vi "Siglent SDG X Series Standard Waveform-APP.vi"() -> ()   [LabVIEW 2020]
doc: "This example shows how to generate a standard waveform."
uses:
  <instrlib>/Siglent SDG X Series/Siglent SDG X Series.lvlib
panel:
  in  "Low Volts":dbl
  in  "High Volts":dbl=5.0
  in  "OK":bool
  in  "Duty Cycle (50.0%)":dbl=98.0 min=20.0 max=99.0 format="%.1g"
  out "Amplitude (1.0 Vpp)":dbl=5.0 format="%#.3f"
  in  "VISA resource name":refnum<visa-resource-name>
  out "DC Offset (0.00 V)":dbl=-2.5
  in  "Frequency (1000 Hz)":dbl=1.0 format="%#.6g"
  in  "Channel (1:Channel 1)":i32(ring)=1 items=["Channel 1"=1, "Channel 2"=2]
  in  "Waveform Function (0: Sine)":u16(ring)=1 items=["Sine", "Square", "Triangle", "DC", "Pulse", "Arb"]
  # "WARNING. RUN ONLY WHEN LASER IS SHUTTERED"
  # "(c) 2017 SIGLENT TECHNOLOGIES CO.,LTD. ALL RIGHTS RESERVED."
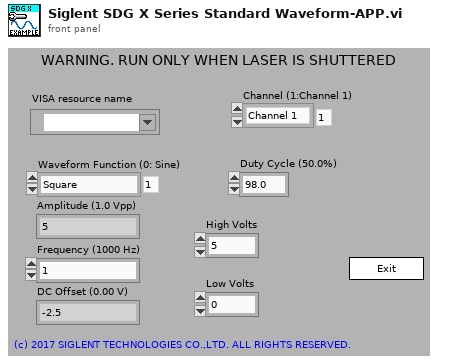
[diagram p1: front panel]
types:
  T1 = enum32{"Invalid", "Standard", "Closed", "Hidden", "Minimized", "Maximized"}
  T2 = enum32{"invalid app kind", "Development System", "Run Time System", "Student Edition", "Embedded LabVIEW", "Evaluation", "Custom"}
  T3 = cluster{"Core":cluster{"Current VI Reference":refnum<vi>, "Close Panel on Exit?":bool}, "VISA resource name":refnum<visa-resource-name>, "Channel (1:Channel 1)":i32}
  T4 = cluster{"Current VI Reference":refnum<vi>, "Close Panel on Exit?":bool}
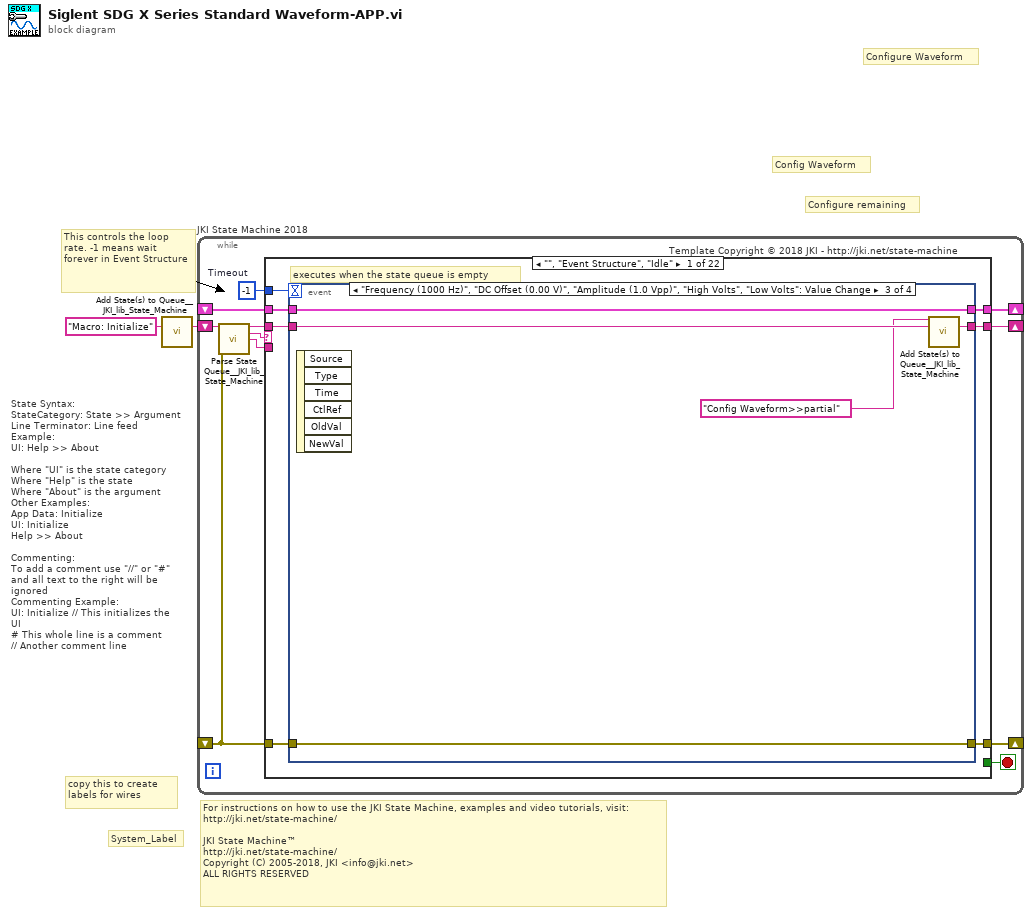
[diagram p0: block diagram]
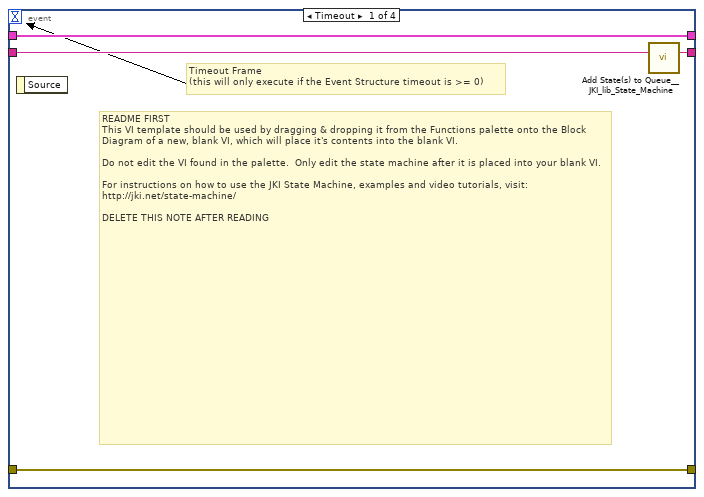
[diagram p2: hidden frame]
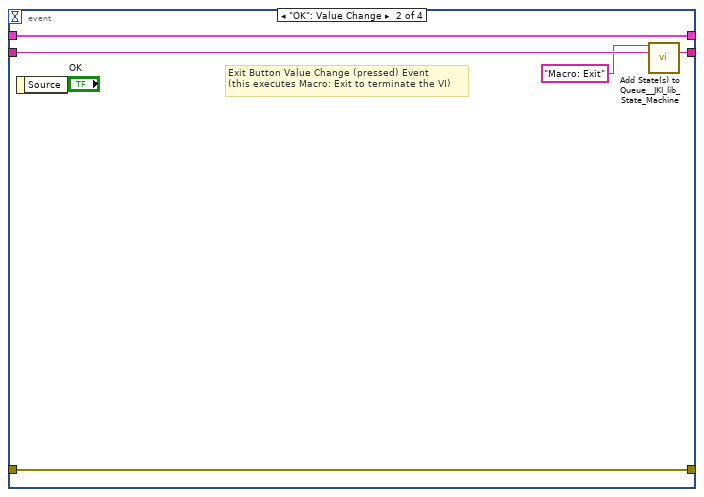
[diagram p3: hidden frame]
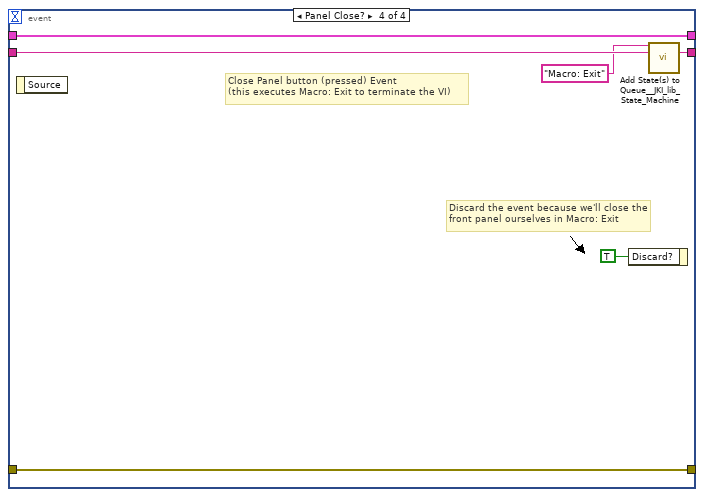
[diagram p4: hidden frame]
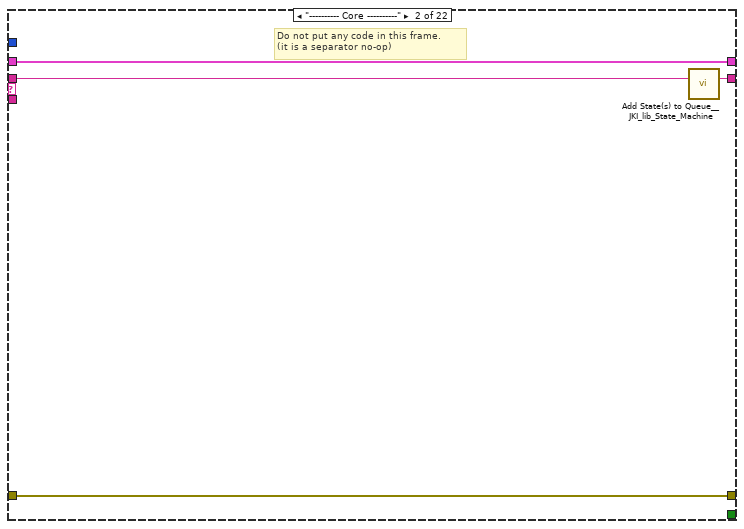
[diagram p5: hidden frame]
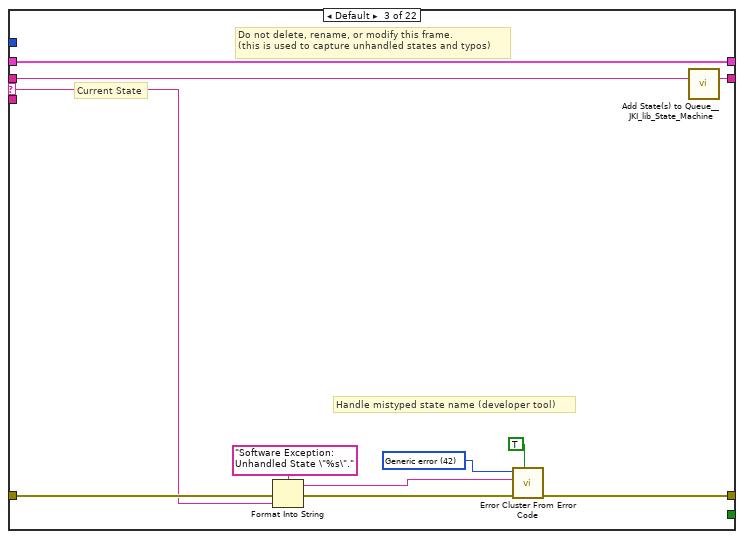
[diagram p6: hidden frame]
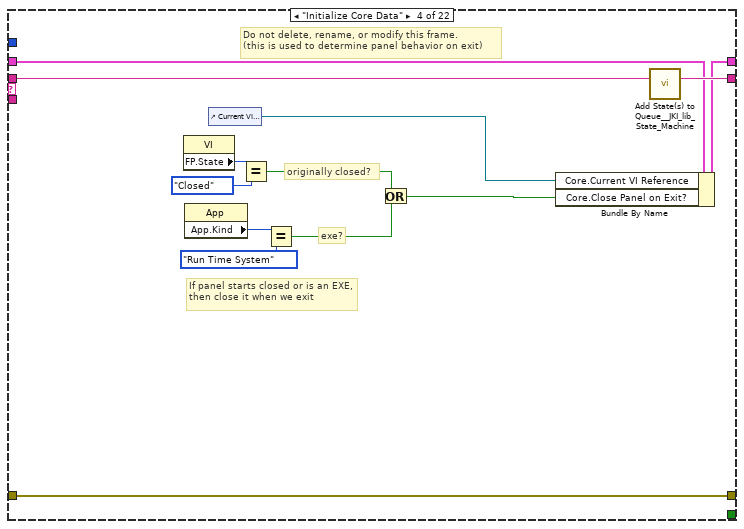
[diagram p7: hidden frame]
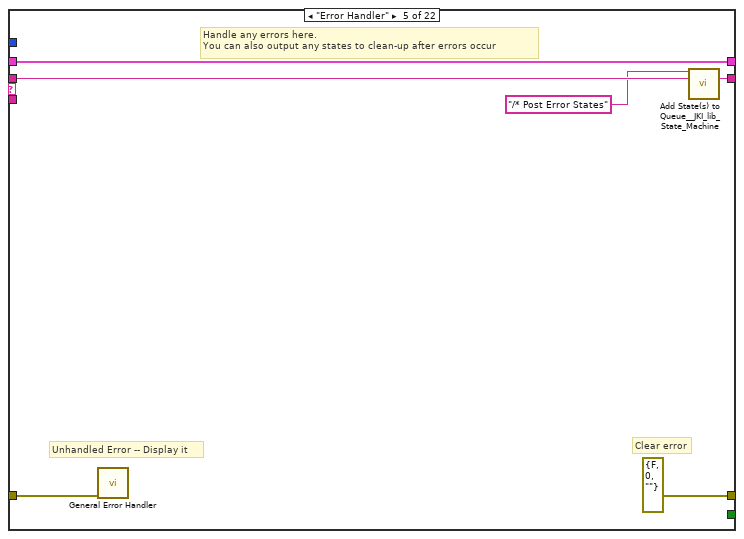
[diagram p8: hidden frame]
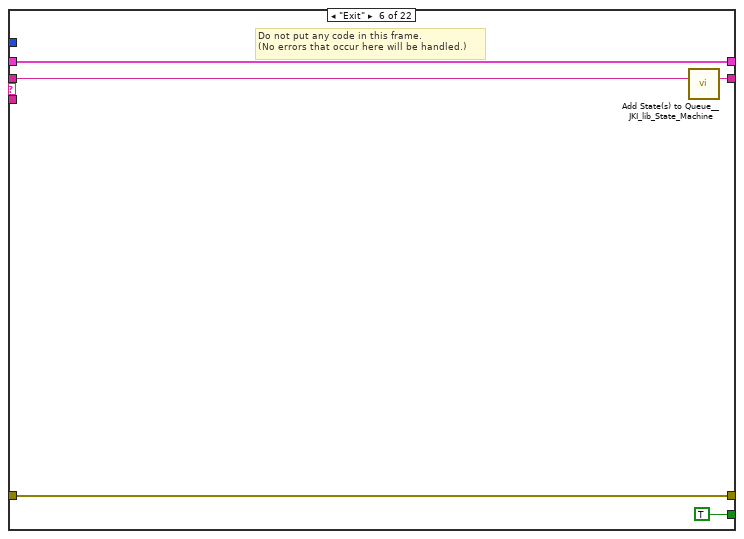
[diagram p9: hidden frame]
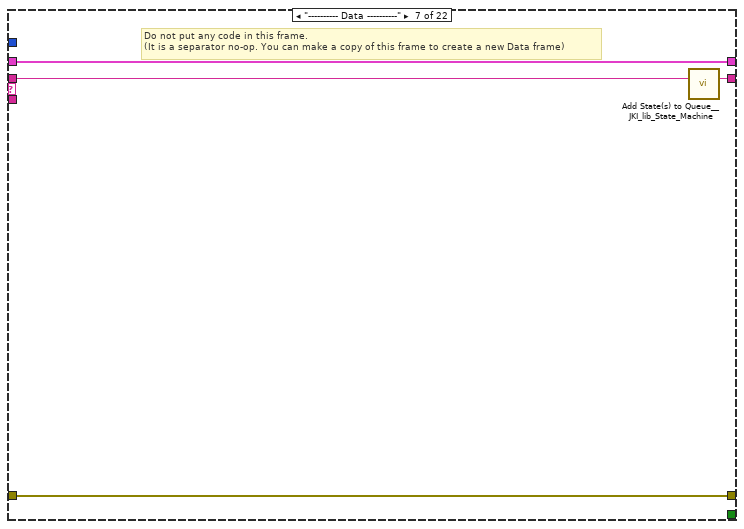
[diagram p10: hidden frame]
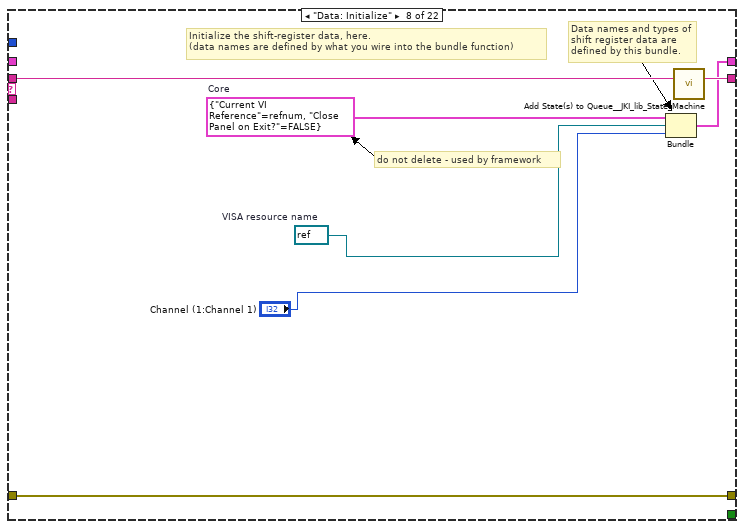
[diagram p11: hidden frame]
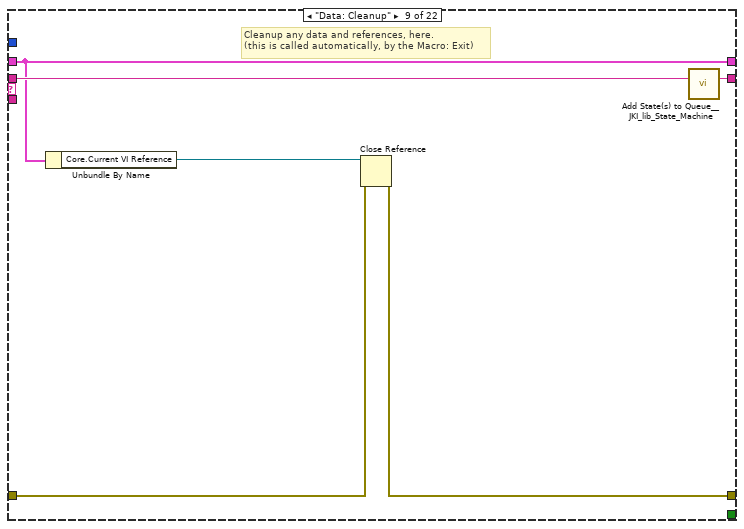
[diagram p12: hidden frame]
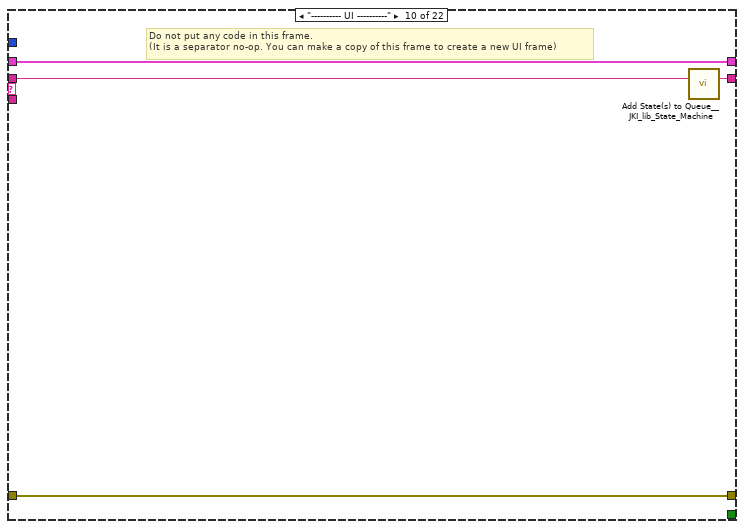
[diagram p13: hidden frame]
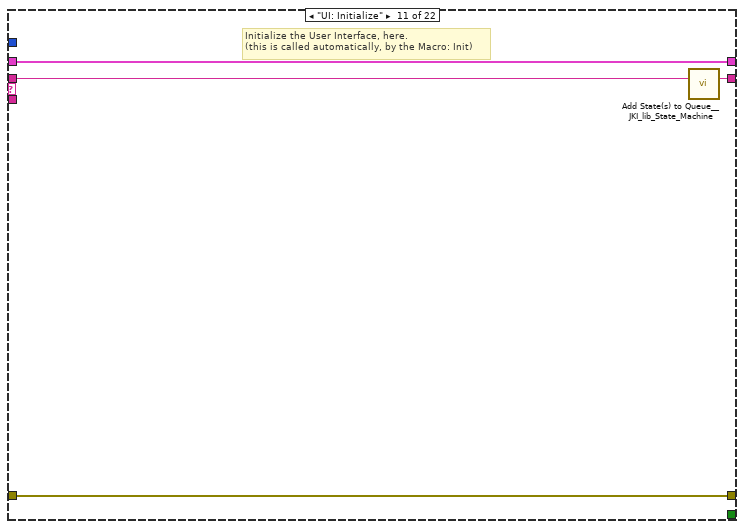
[diagram p14: hidden frame]
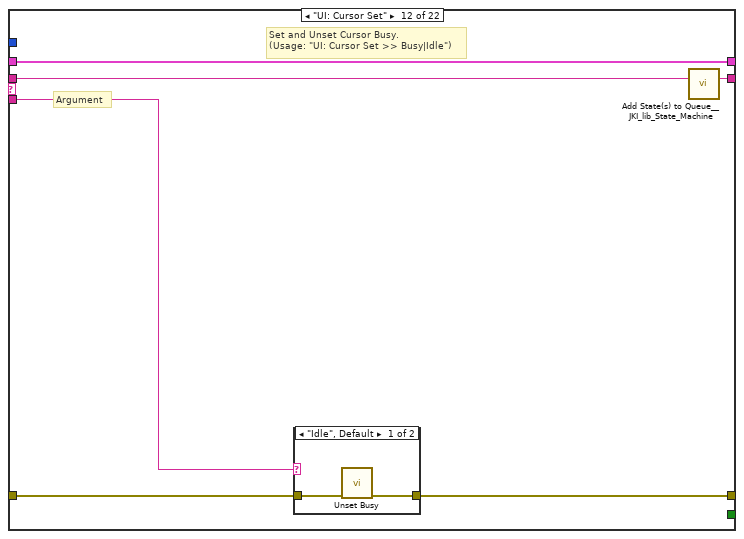
[diagram p15: hidden frame]
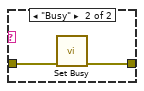
[diagram p16: hidden frame]
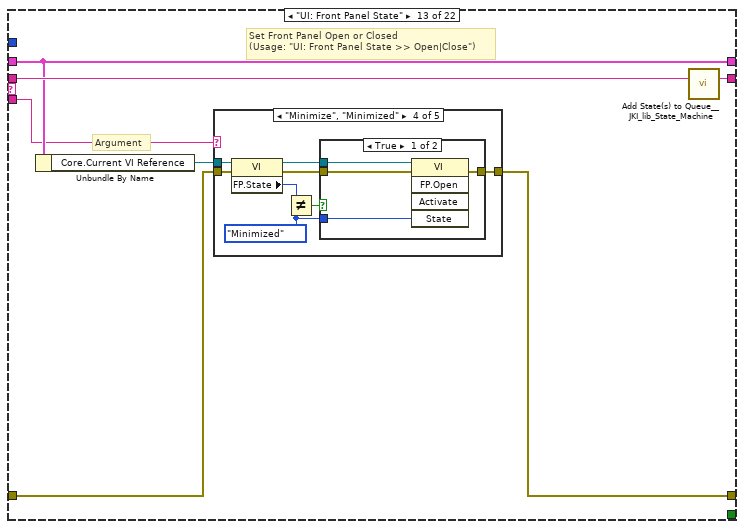
[diagram p17: hidden frame]
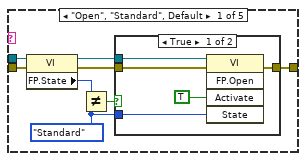
[diagram p18: hidden frame]
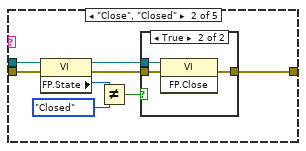
[diagram p20: hidden frame]
diagram:
  # "Configure remaining"
  # "Config Waveform"
  # "For instructions on how to use the JKI State Machine, examples and video tutorials, visit:\nhttp://jki.net/state-machine/\n\nJKI State Machine™\nhttp://jki.net/state-machine/\nCopyright (C) 2005-2018, JKI <info@jki.net>\nALL RIGHTS RESERVED"
  # "State Syntax:\nStateCategory: State >> Argument\nLine Terminator: Line feed\nExample:\nUI: Help >> About\n\nWhere \"UI\" is the state category\nWhere \"Help\" is the state\nWhere \"About\" is the argument\nOther Examples:\nApp Data: Initialize\nUI: Initialize\nHelp >> About\n\nCommenting:\nTo add a comment use \"//\" or \"#\" and all text to the right will be ignored\nCommenting Example:\nUI: Initialize // This initializes the UI\n# This whole line is a comment\n// Another comment line"
  # "copy this to create labels for wires"
  # "This controls the loop rate. -1 means wait forever in Event Structure"
  # "System_Label"
  # "Configure Waveform"
  n1 = call <vilib>:"Add State(s) to Queue__JKI_lib_State_Machine.vi"("State(s) in (\"\")"="Macro: Initialize") -> ("States Out"=w2:string)  [unwired: 14 in]
  n2 = while "JKI State Machine 2018" {
    shift-right: [w6] -> _
    shift-left: _ -> [w5]
    shift-right: [w9] -> _
    shift-left: _ -> [w3]
    shift-right: [w8] -> _
    shift-left: w2 -> [w10]
    stop <- w7 stop-if-true
    w4 = -1  # Timeout
    # "Template Copyright © 2018 JKI - http://jki.net/state-machine"
    n3 = call <vilib>:"Parse State Queue__JKI_lib_State_Machine.vi"("State Queue"=w10, "Error In (no error)"=w3) -> ("Remaining States"=w12:string, "Current State"=w13:string, "Arguments"=w11:string)  [unwired: 11 in]
    n4 = case shown="\"\", \"Event Structure\", \"Idle\"" w13 {
      selector: w13 -> [_ _ w45 _ _ _ _ _ _ _ _ _ _ _ _ _ _ _ _ _ _ _]
      tunnel: w12 -> [w20 w44 w49 w68 w74 w79 w83 w90 w96 w100 w104 w110 w121 w190 w195 w205 w209 w223 w243 w249 w269 w277]
      tunnel: w11 -> [_ _ _ _ _ _ _ _ _ _ _ w105 w115 _ _ _ _ w214 _ _ _ _]
      tunnel: w5 -> [w18 w41 w47 w61 w71 w77 w80 _ w91 w97 w102 w108 w117 w187 w192 w202 w206 w217 w240 w247 w267 w272]
      tunnel: [w17 w42 w51 w65 errorcluster {"status"=FALSE, "code"=0, "source"=""} ("error out") w76 w81 w87 w92 w98 w101 w106 w118 w188 w193 w203 w207 w218 w241 w244 w252 w275] -> w9
      tunnel: w3 -> [w16 w42 w50 w65 w70 w76 w81 w87 w93 w98 w101 w107 w119 w188 w193 w203 w207 w219 w241 w245 w253 w275]
      tunnel: [w19 w43 w48 w67 w73 w78 w82 w89 w95 w99 w103 w109 w120 w189 w194 w204 w208 w222 w242 w248 w268 w276] -> w8
      tunnel: [_ _ _ _ _ TRUE _ _ _ _ _ _ _ _ _ _ _ _ _ _ _ _] -> w7
      tunnel: [w15 w41 w47 w66 w71 w77 w80 w88 w91 w97 w102 w108 w117 w187 w192 w202 w206 w217 w240 w247 w267 w270] -> w6
      tunnel: w4 -> [w14 _ _ _ _ _ _ _ _ _ _ _ _ _ _ _ _ _ _ _ _ _]
      frame "", "Event Structure", "Idle" {
        # "executes when the state queue is empty"
        n5 = event shown="[2] \"Frequency (1000 Hz)\", \"DC Offset (0.00 V)\", \"Amplitude (1.0 Vpp)\", \"High Volts\", \"Low Volts\": Value Change" {
          selector: _ -> [_ _ _ _]
          dyn-events: _ -> [_ _ _ _]
          timeout: w14 -> [_ _ _ _]
          tunnel: w20 -> [w24 w29 w34 w40]
          tunnel: [w23 w28 w33 w39] -> w19
          tunnel: w18 -> [w21 w26 w31 w37]
          tunnel: [w22 w27 w32 w38] -> w17
          tunnel: w16 -> [w22 w27 w32 w38]
          tunnel: [w21 w26 w31 w37] -> w15
          event Timeout {
            # "README FIRST\nThis VI template should be used by dragging & dropping it from the Functions palette onto the Block Diagram of a new, blank VI, which will place it's contents into the blank VI.\n\nDo not edit the VI found in the palette.  Only edit the state machine after it is placed into your blank VI.\n\nFor instructions on how to use the JKI State Machine, examples and video tutorials, visit:\nhttp://jki.net/state-machine/\n\nDELETE THIS NOTE AFTER READING"
            # "Timeout Frame\n(this will only execute if the Event Structure timeout is >= 0)"
            n6 = event-data() -> ()  [unwired: 1 in, 1 out]
            n7 = call <vilib>:"Add State(s) to Queue__JKI_lib_State_Machine.vi"("State(s) in (\"\")"=w24) -> ("States Out"=w23:string)  [unwired: 14 in]
          }
          event "OK": Value Change {
            # "Exit Button Value Change (pressed) Event\n(this executes Macro: Exit to terminate the VI)"
            n8 = event-data() -> ()  [unwired: 1 in, 1 out]
            n9 = call <vilib>:"Add State(s) to Queue__JKI_lib_State_Machine.vi"("State(s) in Front (\"\")"="Macro: Exit", "State(s) in (\"\")"=w29) -> ("States Out"=w28:string)  [unwired: 13 in]
          }
          event "Frequency (1000 Hz)", "DC Offset (0.00 V)", "Amplitude (1.0 Vpp)", "High Volts", "Low Volts": Value Change {
            n10 = event-data() -> ()  [unwired: 1 in, 6 out]
            n11 = call <vilib>:"Add State(s) to Queue__JKI_lib_State_Machine.vi"("State(s) in Front (\"\")"="Config Waveform>>partial", "State(s) in (\"\")"=w34) -> ("States Out"=w33:string)  [unwired: 13 in]
          }
          event Panel Close? {
            # "Discard the event because we'll close the front panel ourselves in Macro: Exit"
            # "Close Panel button (pressed) Event\n(this executes Macro: Exit to terminate the VI)"
            n12 = event-data() -> ()  [unwired: 1 in, 1 out]
            n13 = event-data("Discard?"=TRUE) -> ()  [unwired: 1 in, 1 out]
            n14 = call <vilib>:"Add State(s) to Queue__JKI_lib_State_Machine.vi"("State(s) in Front (\"\")"="Macro: Exit", "State(s) in (\"\")"=w40) -> ("States Out"=w39:string)  [unwired: 13 in]
          }
        }
      }
      frame "---------- Core ----------" {
        # "Do not put any code in this frame.\n(it is a separator no-op)"
        n15 = call <vilib>:"Add State(s) to Queue__JKI_lib_State_Machine.vi"("State(s) in (\"\")"=w44) -> ("States Out"=w43:string)  [unwired: 14 in]
      }
      frame Default {
        w54 = 42 items=["No error", "Argument error", "Memory is full", "Out of zone", "End of file", "File already open", "Generic file I/O error", "File not found", "File permission error", "Disk is full", "Duplicate path", "Too many files open", "System feature not enabled", "Resource file not found", "Cannot add resource", "Resource not found", "Image not found", "Image memory error", "Pen does not exist", "Config type invalid", "Config token not found", "Config parse error", "Config memory error", "Bad external code format", "Bad external code offset", "External code not present", "Null window", "Destroy window error", "Null menu", "Print aborted", "Bad print record", "Print driver error", "Windows error during printing", "Memory error during printing", "Print dialog error", "Generic print error", "Invalid device refnum", "Device not found", "Device parameter error", "Device unit error", "Cannot open device", "Device call aborted", "Generic error", "Cancelled by user", "Object ID too low", "Object ID too high", "Object not in heap", "Unknown heap", "Unknown object (invalid DefProc)", "Unknown object (DefProc not in table)", "Message out of range", "Invalid (null) method", "Unknown message", "Manager call not supported", "Bad address", "Network operation in progress", "Network operation timed out", "Connection is busy", "Network attribute not supported", "Network error", "Address in use", "System out of memory", "Connection aborted", "Connection refused", "Not connected", "Already connected", "Connection closed", "Initialization error (interapplication manager)", "Bad occurrence", "Wait on unbound occurrence handler", "Occurrence queue overflow", "Datalog type conflict", "Unused", "Unrecognized type (interapplication manager)", "Memory corrupt", "Failed to make temporary DLL", "Old CIN version", "Drag socket not found", "Failed to load drop-object", "Failed to register OLE object", "Failed to release OLE object", "Format specifier type mismatch", "Unknown format specifier", "Too few format specifiers", "Too many format specifiers", "Scan failed", "Newer CIN version", "Error converting to variant", "Runtime menu error", "Password tampered", "Variant attribute not found", "Incompatible variant data type", "Event data is not available", "Event Store is not present", "Occurrence is not found", "Event Queue is not created", "Event info is not available", "Refnum passed is NULL", "Error retrieving Class GUID", "Error retrieving CoClass GUID", "Error retrieving TypeLib GUID.", "Bad built application magic bytes.", "Specific driver is different from the specific driver associated with the Logical Name.", "There is no session opened to the class driver.", "Max Error", "MAX - Error with config objects", "MAX - Error loading configuration", "MAX - Group not supported"]
        # "Current State"
        # "Do not delete, rename, or modify this frame.\n(this is used to capture unhandled states and typos)"
        # "Handle mistyped state name (developer tool)"
        n16 = Format Into String(format string="Software Exception: Unhandled State \"%s\"." ("message"), error in=w50, w45) -> (resulting string=w53:string, error out=w52:errorcluster)  [unwired: 1 in]
        n17 = call <vilib>:"Error Cluster From Error Code.vi"("show call chain? (False)"=TRUE, "error in (no error)"=w52, "error message (\"\")"=w53, "error code (0)"=w54) -> ("error out"=w51:errorcluster)  [unwired: 5 in]
        n18 = call <vilib>:"Add State(s) to Queue__JKI_lib_State_Machine.vi"("State(s) in (\"\")"=w49) -> ("States Out"=w48:string)  [unwired: 14 in]
      }
      frame "Initialize Core Data" {
        # "Do not delete, rename, or modify this frame.\n(this is used to determine panel behavior on exit)"
        # "originally closed?"
        # "exe?"
        # "If panel starts closed or is an EXE, then close it when we exit"
        n19 = property class="VI"() -> ("FP.State"=w58:T1)  [unwired: 2 in, 2 out]
        n20 = property class="App"() -> ("App.Kind"=w64:T2)  [unwired: 2 in, 2 out]
        n21 = control-ref of="Current VI Reference"() -> (w59:refnum<vi>)
        n22 = Equal?(x=w58, y=T1."Closed" ("Front Panel Window:State")) -> (x = y?=w56:bool)
        n23 = Equal?(x=w64, y=T2."Run Time System" ("Application:Kind")) -> (x = y?=w62:bool)
        n24 = Or(x=w56, y=w62) -> (x .or. y?=w60:bool)
        n25 = Bundle By Name(cluster=w61, "Core.Current VI Reference"=w59, "Core.Close Panel on Exit?"=w60) -> (w66:T3)
        n26 = call <vilib>:"Add State(s) to Queue__JKI_lib_State_Machine.vi"("State(s) in (\"\")"=w68) -> ("States Out"=w67:string)  [unwired: 14 in]
      }
      frame "Error Handler" {
        # "Unhandled Error -- Display it"
        # "Handle any errors here.\nYou can also output any states to clean-up after errors occur"
        # "Clear error"
        n27 = call <vilib>:"General Error Handler.vi"("error in (no error)"=w70) -> ()  [unwired: 10 in, 5 out]
        n28 = call <vilib>:"Add State(s) to Queue__JKI_lib_State_Machine.vi"("State(s) in Front (\"\")"="/* Post Error States", "State(s) in (\"\")"=w74) -> ("States Out"=w73:string)  [unwired: 13 in]
      }
      frame "Exit" {
        # "Do not put any code in this frame.\n(No errors that occur here will be handled.)"
        n29 = call <vilib>:"Add State(s) to Queue__JKI_lib_State_Machine.vi"("State(s) in (\"\")"=w79) -> ("States Out"=w78:string)  [unwired: 14 in]
      }
      frame "---------- Data ----------" {
        # "Do not put any code in this frame.\n(It is a separator no-op. You can make a copy of this frame to create a new Data frame)"
        n30 = call <vilib>:"Add State(s) to Queue__JKI_lib_State_Machine.vi"("State(s) in (\"\")"=w83) -> ("States Out"=w82:string)  [unwired: 14 in]
      }
      frame "Data: Initialize" {
        w85 = refnum<visa-resource-name> refnum  # VISA resource name
        w86 = T4 {"Current VI Reference"=refnum, "Close Panel on Exit?"=FALSE}  # Core
        # "do not delete - used by framework"
        # "Data names and types of shift register data are defined by this bundle."
        # "Initialize the shift-register data, here.\n(data names are defined by what you wire into the bundle function)"
        n31 = Bundle("Core"=w86, "VISA resource name"=w85, "Channel (1:Channel 1)"="Channel (1:Channel 1)") -> (w88:T3)  [unwired: 1 in]
        n32 = call <vilib>:"Add State(s) to Queue__JKI_lib_State_Machine.vi"("State(s) in (\"\")"=w90) -> ("States Out"=w89:string)  [unwired: 14 in]
      }
      frame "Data: Cleanup" {
        # "Cleanup any data and references, here.\n(this is called automatically, by the Macro: Exit)"
        n33 = Unbundle By Name(w91) -> ("Core.Current VI Reference"=w94:refnum<vi>)
        n34 = Close Reference(reference=w94, error in (no error)=w93) -> (error out=w92:errorcluster)
        n35 = call <vilib>:"Add State(s) to Queue__JKI_lib_State_Machine.vi"("State(s) in (\"\")"=w96) -> ("States Out"=w95:string)  [unwired: 14 in]
      }
      frame "---------- UI ----------" {
        # "Do not put any code in this frame.\n(It is a separator no-op. You can make a copy of this frame to create a new UI frame)"
        n36 = call <vilib>:"Add State(s) to Queue__JKI_lib_State_Machine.vi"("State(s) in (\"\")"=w100) -> ("States Out"=w99:string)  [unwired: 14 in]
      }
      frame "UI: Initialize" {
        # "Initialize the User Interface, here.\n(this is called automatically, by the Macro: Init)"
        n37 = call <vilib>:"Add State(s) to Queue__JKI_lib_State_Machine.vi"("State(s) in (\"\")"=w104) -> ("States Out"=w103:string)  [unwired: 14 in]
      }
      frame "UI: Cursor Set" {
        # "Argument"
        # "Set and Unset Cursor Busy.\n(Usage: \"UI: Cursor Set >> Busy|Idle\")"
        n38 = case shown="\"Idle\", Default" w105 {
          tunnel: w107 -> [w112 w114]
          tunnel: [w111 w113] -> w106
          frame "Idle", Default {
            n39 = call <vilib>:"Unset Busy.vi"("error in (no error)"=w112) -> ("error out"=w111:errorcluster)  [unwired: 10 in]
          }
          frame "Busy" {
            n40 = call <vilib>:"Set Busy.vi"("error in (no error)"=w114) -> ("error out"=w113:errorcluster)  [unwired: 9 in, 1 out]
          }
        }
        n41 = call <vilib>:"Add State(s) to Queue__JKI_lib_State_Machine.vi"("State(s) in (\"\")"=w110) -> ("States Out"=w109:string)  [unwired: 14 in]
      }
      frame "UI: Front Panel State" {
        # "Argument"
        # "Set Front Panel Open or Closed\n(Usage: \"UI: Front Panel State >> Open|Close\")"
        n42 = Unbundle By Name(w117) -> ("Core.Current VI Reference"=w116:refnum<vi>)
        n43 = case shown="\"Minimize\", \"Minimized\"" w115 {
          tunnel: w119 -> [w127 w142 w153 w166 w179]
          tunnel: [w129 w143 w155 w168 w181] -> w118
          tunnel: w116 -> [w128 w140 w154 w167 w180]
          frame "Open", "Standard", Default {
            w122 = T1."Standard" ("State")
            n44 = property class="VI"(reference=w128, error in=w127) -> (reference out=w125:refnum<vi>, error out=w126:errorcluster, "FP.State"=w124:T1)
            n45 = Not Equal?(x=w124, y=w122) -> (x != y?=w123:bool)
            n46 = case shown="True" w123 {
              tunnel: [w133 w135] -> w129
              tunnel: w126 -> [w132 w135]
              tunnel: w125 -> [w131 _]
              tunnel: w122 -> [w130 _]
              frame True {
                n47 = invoke class="VI" method="FP.Open"(reference=w131, error in=w132, "Activate"=TRUE, "State"=w130) -> (error out=w133:errorcluster)  [unwired: 1 in, 4 out]
              }
              frame False {
              }
            }
          }
          frame "Close", "Closed" {
            n48 = property class="VI"(reference=w140, error in=w142) -> (reference out=w139:refnum<vi>, error out=w141:errorcluster, "FP.State"=w137:T1)
            n49 = Not Equal?(x=w137, y=T1."Closed" ("Front Panel Window:State")) -> (x != y?=w136:bool)
            n50 = case shown="True" w136 {
              tunnel: [w144 w147] -> w143
              tunnel: w141 -> [w144 w146]
              tunnel: w139 -> [_ w145]
              frame False {
              }
              frame True {
                n51 = invoke class="VI" method="FP.Close"(reference=w145, error in=w146) -> (error out=w147:errorcluster)  [unwired: 1 in, 2 out]
              }
            }
          }
          frame "Hidden", "Hide" {
            w148 = T1."Hidden" ("State")
            n52 = property class="VI"(reference=w154, error in=w153) -> (reference out=w151:refnum<vi>, error out=w152:errorcluster, "FP.State"=w150:T1)
            n53 = Not Equal?(x=w150, y=w148) -> (x != y?=w149:bool)
            n54 = case shown="True" w149 {
              tunnel: [w159 w160] -> w155
              tunnel: w152 -> [w158 w160]
              tunnel: w151 -> [w157 _]
              tunnel: w148 -> [w156 _]
              frame True {
                n55 = invoke class="VI" method="FP.Open"(reference=w157, error in=w158, "State"=w156) -> (error out=w159:errorcluster)  [unwired: 2 in, 4 out]
              }
              frame False {
              }
            }
          }
          frame "Minimize", "Minimized" {
            w161 = T1."Minimized" ("State")
            n56 = property class="VI"(reference=w167, error in=w166) -> (reference out=w164:refnum<vi>, error out=w165:errorcluster, "FP.State"=w163:T1)
            n57 = Not Equal?(x=w163, y=w161) -> (x != y?=w162:bool)
            n58 = case shown="True" w162 {
              tunnel: [w172 w173] -> w168
              tunnel: w165 -> [w171 w173]
              tunnel: w164 -> [w170 _]
              tunnel: w161 -> [w169 _]
              frame True {
                n59 = invoke class="VI" method="FP.Open"(reference=w170, error in=w171, "State"=w169) -> (error out=w172:errorcluster)  [unwired: 2 in, 4 out]
              }
              frame False {
              }
            }
          }
          frame "Maximize", "Maximized" {
            w174 = T1."Maximized" ("State")
            n60 = property class="VI"(reference=w180, error in=w179) -> (reference out=w177:refnum<vi>, error out=w178:errorcluster, "FP.State"=w176:T1)
            n61 = Not Equal?(x=w176, y=w174) -> (x != y?=w175:bool)
            n62 = case shown="True" w175 {
              tunnel: [w185 w186] -> w181
              tunnel: w178 -> [w184 w186]
              tunnel: w177 -> [w183 _]
              tunnel: w174 -> [w182 _]
              frame True {
                n63 = invoke class="VI" method="FP.Open"(reference=w183, error in=w184, "State"=w182) -> (error out=w185:errorcluster)  [unwired: 2 in, 4 out]
              }
              frame False {
              }
            }
          }
        }
        n64 = call <vilib>:"Add State(s) to Queue__JKI_lib_State_Machine.vi"("State(s) in (\"\")"=w121) -> ("States Out"=w120:string)  [unwired: 14 in]
      }
      frame "---------- Macro ----------" {
        # "Do not put any code in this frame.\n(It is a separator no-op. You can make a copy of this frame to create a new Macro frame)"
        n65 = call <vilib>:"Add State(s) to Queue__JKI_lib_State_Machine.vi"("State(s) in (\"\")"=w190) -> ("States Out"=w189:string)  [unwired: 14 in]
      }
      frame "Macro: Initialize" {
        # "Initialization Macro\n(This is called once, when the VI starts)"
        n66 = call <vilib>:"Add State(s) to Queue__JKI_lib_State_Machine.vi"("State(s) in Front (\"\")"="Data: Initialize\nInitialize Core Data\nUI: Initialize\nUI: Front Panel State >> Open\nInit\nConfig Waveform\nConfigure remaining", "State(s) in (\"\")"=w195) -> ("States Out"=w194:string)  [unwired: 13 in]
      }
      frame "Macro: Exit" {
        # "Exit Macro\n(This is called once, when the VI exits)"
        n67 = Unbundle By Name(w202) -> ("Core.Close Panel on Exit?"=w201:bool)
        n68 = Select(t="UI: Front Panel State >> Close", s=w201, f="") -> (s? t:f=w198:string)
        n69 = call <vilib>:"Add State(s) to Queue__JKI_lib_State_Machine.vi"("State(s) in (\"\")"=w198, "State(s) at Back (\"\")"="close\nData: Cleanup\nExit") -> ("States Out"=w196:string)  [unwired: 13 in]
        n70 = call <vilib>:"Add State(s) to Queue__JKI_lib_State_Machine.vi"("State(s) in Front (\"\")"=w196, "State(s) in (\"\")"=w205) -> ("States Out"=w204:string)  [unwired: 13 in]
      }
      frame "---------- New Category ----------" {
        n71 = call <vilib>:"Add State(s) to Queue__JKI_lib_State_Machine.vi"("State(s) in (\"\")"=w209) -> ("States Out"=w208:string)  [unwired: 14 in]
      }
      frame "Config Waveform" {
        n72 = Unbundle By Name(w217) -> ("VISA resource name"=w216:refnum<visa-resource-name>, "Channel (1:Channel 1)"=w215:i32)
        n73 = call "volts to amp offset.vi"("Low Volts"="Low Volts", "High Volts"="High Volts") -> ("DC Offset (0.00 V)"=w213:dbl, "Amplitude (1.0 Vpp)"=w210:dbl)  [unwired: 8 in]
        "DC Offset (0.00 V)" <- w213
        "Amplitude (1.0 Vpp)" <- w210
        n74 = case shown="\"partial\"" w214 {
          tunnel: w210 -> [w231 w239]
          tunnel: w213 -> [w230 w238]
          tunnel: "Frequency (1000 Hz)" -> [w229 w237]
          tunnel: "Waveform Function (0: Sine)" -> [w228 w236]
          tunnel: w219 -> [w227 w235]
          tunnel: [w226 w234] -> w218
          tunnel: w216 -> [w225 w233]
          tunnel: w215 -> [w224 w232]
          frame "True", Default {
            n75 = call <instrlib>:"Configure Standard Waveform.vi"("VISA resource name"=w225, "Waveform Function (0: Sine)"=w228, "Channel (1:Channel 1)"=w224, "Amplitude (1.0 Vpp)"=w231, "Frequency (1000 Hz)"=w229, "DC Offset (0.00 V)"=w230, "error in (no error)"=w227) -> ("error out"=w226:errorcluster)  [unwired: 7 in, 1 out]
          }
          frame "partial" {
            n76 = call "Configure Standard Waveform Amplitude and Offset.vi"("VISA resource name"=w233, "Waveform Function (0: Sine)"=w236, "Channel (1:Channel 1)"=w232, "Amplitude (1.0 Vpp)"=w239, "Frequency (1000 Hz)"=w237, "DC Offset (0.00 V)"=w238, "error in (no error)"=w235) -> ("error out"=w234:errorcluster)  [unwired: 7 in, 1 out]
          }
        }
        n77 = call <vilib>:"Add State(s) to Queue__JKI_lib_State_Machine.vi"("State(s) in (\"\")"=w223) -> ("States Out"=w222:string)  [unwired: 14 in]
      }
      frame "New Category: 2" {
        n78 = Unbundle By Name(w240) -> ()  [unwired: 2 out]
        n79 = call <vilib>:"Add State(s) to Queue__JKI_lib_State_Machine.vi"("State(s) in (\"\")"=w243) -> ("States Out"=w242:string)  [unwired: 14 in]
      }
      frame "close" {
        n80 = Unbundle By Name(w247) -> ("VISA resource name"=w246:refnum<visa-resource-name>)  [unwired: 1 out]
        n81 = call <instrlib>:"Close.vi"("error in (no error)"=w245, "VISA resource name"=w246) -> ("error out"=w244:errorcluster)  [unwired: 9 in]
        n82 = call <vilib>:"Add State(s) to Queue__JKI_lib_State_Machine.vi"("State(s) in (\"\")"=w249) -> ("States Out"=w248:string)  [unwired: 14 in]
      }
      frame "Configure remaining" {
        w258 = u16 0 items=["N-Cycle", "Infinite"] ("Burst Cycle (0: N-Cycle)")
        w256 = u16 1 items=["Internal", "External", "Manual"] ("Trigger Source (0: Internal)")
        w254 = TRUE  # Enable Output
        # "Enable Output"
        n83 = Unbundle By Name(w267) -> ("VISA resource name"=w251:refnum<visa-resource-name>, "Channel (1:Channel 1)"=w250:i32)
        n84 = call <instrlib>:"Configure Burst.vi"("VISA resource name"=w251, "Burst Cycle (0: N-Cycle)"=w258, "Number of Cycles (1)"=1, "error in (no error)"=w253, "Trigger Source (0: Internal)"=w256, "Enable Burst Mode (T:Enable)"=TRUE, "Channel (1:Channel 1)"=w250) -> ("VISA resource name out"=w262:refnum<visa-resource-name>, "error out"=w261:errorcluster)  [unwired: 11 in]
        n85 = call <instrlib>:"Configure Duty Cycle.vi"("error in (no error)"=w261, "Duty Cycle (50.0%)"="Duty Cycle (50.0%)", "Channel (1:Channel 1)"=w250, "VISA resource name"=w262) -> ("error out"=w265:errorcluster, "VISA resource name out"=w263:refnum<visa-resource-name>)  [unwired: 6 in]
        n86 = call <instrlib>:"Invert Output.vi"("error in (no error)"=w265, "Enable Channel Invert (F: Disable)"=TRUE, "Channel (1:Channel 1)"=w250, "VISA resource name"=w263) -> ("error out"=w266:errorcluster, "VISA resource name out"=w264:refnum<visa-resource-name>)  [unwired: 6 in]
        n87 = call <instrlib>:"Enable Output.vi"("error in (no error)"=w266, "Enable Output (T: Enable)"=w254, "Channel (1:Channel 1)"=w250, "VISA resource name"=w264) -> ("error out"=w252:errorcluster)  [unwired: 6 in, 1 out]
        n88 = call <vilib>:"Add State(s) to Queue__JKI_lib_State_Machine.vi"("State(s) in (\"\")"=w269) -> ("States Out"=w268:string)  [unwired: 14 in]
      }
      frame "Init" {
        n89 = call <instrlib>:"Initialize.vi"("Reset (True)"=FALSE, "VISA resource name"="VISA resource name") -> ("VISA resource name out"=w271:refnum<visa-resource-name>)  [unwired: 8 in, 1 out]
        n90 = Bundle By Name(cluster=w272, "VISA resource name"=w271) -> (w270:T3)
        n91 = call <vilib>:"Add State(s) to Queue__JKI_lib_State_Machine.vi"("State(s) in (\"\")"=w277) -> ("States Out"=w276:string)  [unwired: 14 in]
      }
    }
  }
